vi "Simple RT Add.vi"(8 "error in (no error)":errorcluster, 9 "y":dbl, 10 "x":dbl) -> (0 "error out":errorcluster, 2 "x+y":dbl)   [LabVIEW 2018]
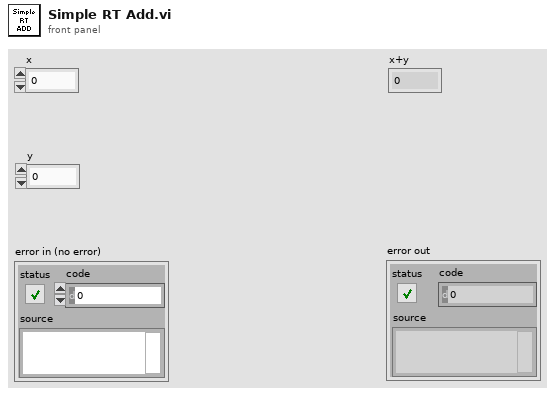
[diagram p1: front panel]
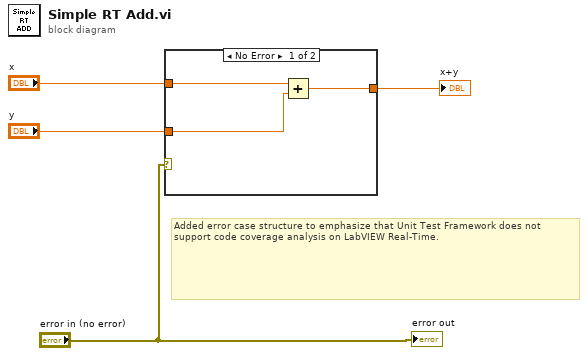
[diagram p0: block diagram]
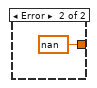
[diagram p2: hidden frame]
diagram:
  # "Added error case structure to emphasize that Unit Test Framework does not support code coverage analysis on LabVIEW Real-Time."
  n1 = case shown="No Error" "error in (no error)" {
    tunnel: "y" -> [w7 _]
    tunnel: "x" -> [w6 _]
    tunnel: [w5 nan] -> w2
    frame No Error {
      n2 = Add(x=w6, y=w7) -> (x+y=w5:dbl)
    }
    frame Error {
    }
  }
  "x+y" <- w2
  "error out" <- "error in (no error)"
